vi "Gaussian_point_spacing.vi"(0 "Start point":dbl format="%.2f", 1 "No of points":i32, 2 "Centre point":dbl format="%.2f", 3 "End point":dbl format="%.2f", 4 "Guass intensity":dbl=1.5 min=0.01 format="%.4f") -> (5 "Positions":dbl[](array[numeric]) format="%.2f")   [LabVIEW 2012]
uses:
  <vilib>/Analysis/NI_AALPro.lvlib
panel:
  out "?":cluster{dbl[], dbl[]}(graph)
  out "Sigma":dbl format="%.2f"
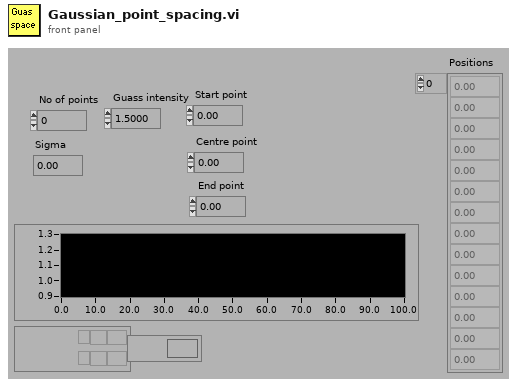
[diagram p1: front panel]
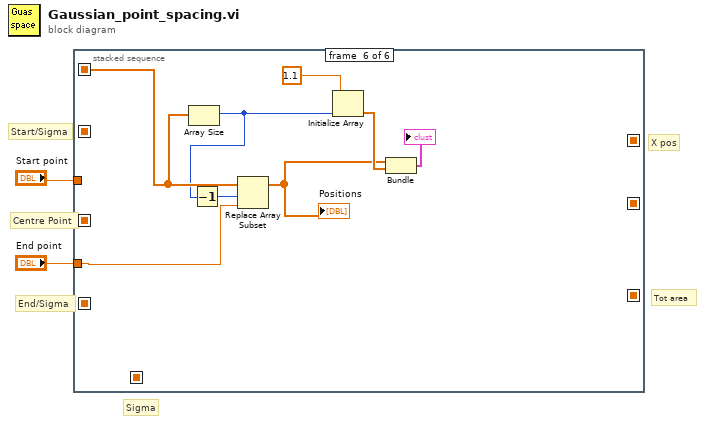
[diagram p0: block diagram]
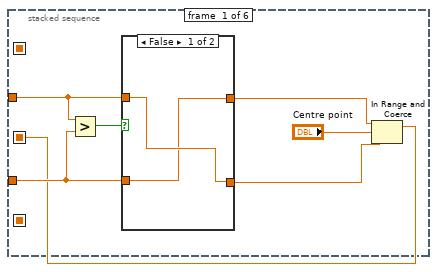
[diagram p2: hidden frame]
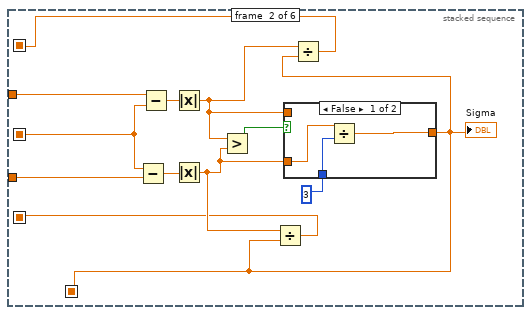
[diagram p4: hidden frame]
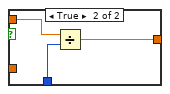
[diagram p5: hidden frame]
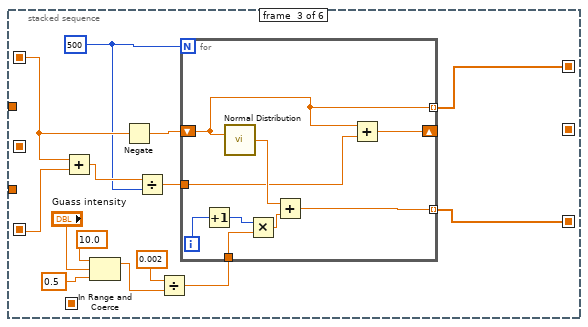
[diagram p6: hidden frame]
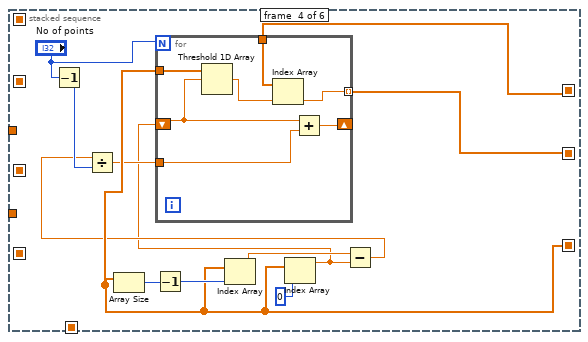
[diagram p7: hidden frame]
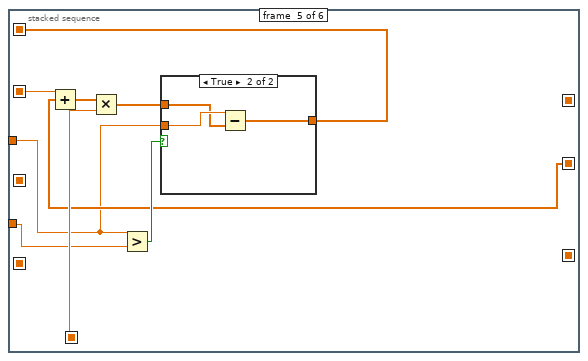
[diagram p8: hidden frame]
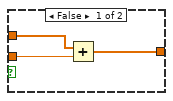
[diagram p9: hidden frame]
diagram:
  # "Centre Point"
  # "End/Sigma"
  # "Start/Sigma"
  # "Sigma"
  # "Tot area"
  # "X pos"
  n1 = stacked-sequence {
    seq-local: [_ _ w45 _ _ _] -> [_ _ _ w64 _ _]
    seq-local: [_ _ w44 _ _ _] -> [_ _ _ w60 _ _]
    seq-local: [_ w18 _ _ _ _] -> [_ _ _ _ w81 _]
    seq-local: [_ w20 _ _ _ _] -> [_ _ w41 _ w82 _]
    seq-local: [_ w17 _ _ _ _] -> [_ _ w43 _ _ _]
    seq-local: [_ _ _ w63 _ _] -> [_ _ _ _ w76 _]
    seq-local: [_ _ _ _ w74 _] -> [_ _ _ _ _ w93]
    seq-local: [w3 _ _ _ _ _] -> [_ w14 _ _ _ _]
    tunnel: "Start point" -> [w6 w15 _ _ w75 _]
    tunnel: "End point" -> [w4 w16 _ _ w79 w91]
    frame #0 {
      n2 = Greater?(x=w6, y=w4) -> (0:w8:bool)
      n3 = case shown="False" w8 {
        tunnel: [w10 w13] -> w7
        tunnel: w6 -> [w11 w13]
        tunnel: [w11 w12] -> w5
        tunnel: w4 -> [w10 w12]
        frame False {
        }
        frame True {
        }
      }
      n4 = In Range and Coerce(upper limit=w7, x="Centre point", lower limit=w5) -> (coerced(x)=w3:dbl)  [unwired: 1 out]
    }
    frame #1 {
      n5 = Subtract(x=w14, y=w16) -> (x-y=w24:dbl)
      n6 = Subtract(x=w15, y=w14) -> (x-y=w25:dbl)
      n7 = Absolute Value(x=w25) -> (abs(x)=w21:dbl)
      n8 = Absolute Value(x=w24) -> (abs(x)=w19:dbl)
      n9 = Greater?(x=w21, y=w19) -> (0:w23:bool)
      n10 = case shown="False" w23 {
        tunnel: 3 -> [w28 w31]
        tunnel: w21 -> [_ w30]
        tunnel: [w27 w29] -> w18
        tunnel: w19 -> [w26 _]
        frame False {
          n11 = Divide(x=w26, y=w28) -> (x/y=w27:dbl)
        }
        frame True {
          n12 = Divide(x=w30, y=w31) -> (x/y=w29:dbl)
        }
      }
      "Sigma" <- w18
      n13 = Divide(x=w19, y=w18) -> (x/y=w17:dbl)
      n14 = Divide(x=w21, y=w18) -> (x/y=w20:dbl)
    }
    frame #2 {
      w39 = 500
      n15 = Add(x=w41, y=w43) -> (x+y=w40:dbl)
      n16 = In Range and Coerce(upper limit=10.0 ("Max"), x="Guass intensity", lower limit=0.5 ("Min")) -> (coerced(x)=w32:dbl)  [unwired: 1 out]
      n17 = Negate(x=w41) -> (-x=w42:dbl)
      n18 = Divide(x=w40, y=w39) -> (x/y=w38:dbl)
      n19 = Divide(x=0.002, y=w32) -> (x/y=w37:dbl)
      n20 = for {
        N: w39 -> [_]
        shift-right: [w54] -> _
        shift-left: w42 -> [w48]
        tunnel: w37 -> [w50]
        tunnel: [w48] -> w45 mode=indexing
        tunnel: [w52] -> w44 mode=indexing
        tunnel: w38 -> [w51]
        i -> [w47]
        n21 = Increment(x=w47) -> (x+1=w46:i32)
        n22 = call <vilib>:"Normal Distribution.vi"("x"=w48) -> ("probability"=w53:dbl)
        n23 = Multiply(x=w46, y=w50) -> (x*y=w49:dbl)
        n24 = Add(x=w53, y=w49) -> (x+y=w52:dbl)
        n25 = Add(x=w48, y=w51) -> (x+y=w54:dbl)
      }
    }
    frame #3 {
      n26 = Decrement(x="No of points") -> (x-1=w62:i32)
      n27 = Array Size(array=w60) -> (size(s)=w66:i32)
      n28 = Decrement(x=w66) -> (x-1=w65:i32)
      n29 = Index Array(array=w60, index=w65) -> (element=w59:dbl)
      n30 = Index Array(array=w60, index=0) -> (element=w55:dbl)
      n31 = Subtract(x=w59, y=w55) -> (x-y=w58:dbl)
      n32 = Divide(x=w58, y=w62) -> (x/y=w57:dbl)
      n33 = for {
        N: "No of points" -> [_]
        shift-right: [w72] -> _
        shift-left: w55 -> [w67]
        tunnel: w57 -> [w73]
        tunnel: w60 -> [w71]
        tunnel: w64 -> [w70]
        tunnel: [w68] -> w63 mode=indexing
        n34 = Threshold 1D Array(2:w67, 3:w71) -> (0:w69:dbl)  [unwired: 1 out]
        n35 = Index Array(array=w70, index=w69) -> (element=w68:dbl)
        n36 = Add(x=w67, y=w73) -> (x+y=w72:dbl)
      }
    }
    frame #4 {
      n37 = Add(x=w82, y=w76) -> (x+y=w80:dbl[])
      n38 = Multiply(x=w80, y=w81) -> (x*y=w77:dbl[])
      n39 = Greater?(x=w75, y=w79) -> (0:w78:bool)
      n40 = case shown="True" w78 {
        tunnel: w77 -> [w85 w86]
        tunnel: w75 -> [w84 w87]
        tunnel: [w83 w88] -> w74
        frame False {
          n41 = Add(x=w85, y=w84) -> (x+y=w83:dbl[])
        }
        frame True {
          n42 = Subtract(x=w87, y=w86) -> (x-y=w88:dbl[])
        }
      }
    }
    frame #5 {
      n43 = Array Size(array=w93) -> (size(s)=w92:i32)
      n44 = Decrement(x=w92) -> (x-1=w90:i32)
      n45 = Replace Array Subset(array=w93, new element=w91, index=w90) -> (w89:dbl[])
      "Positions" <- w89
      n46 = Initialize Array(1.1, w92) -> (w95:dbl[])
      n47 = Bundle(w89, w95) -> (→"?":cluster{dbl[], dbl[]})  [unwired: 1 out]
    }
  }
